vi "SVN_ParseRevisionNumber.vi"(11 "rev str (In)":string) -> (3 "number":i32)   [LabVIEW 2014]
panel:
  out "offset past number":i32
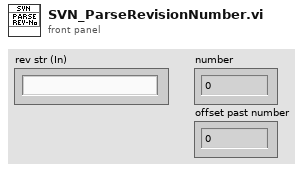
[diagram p1: front panel]
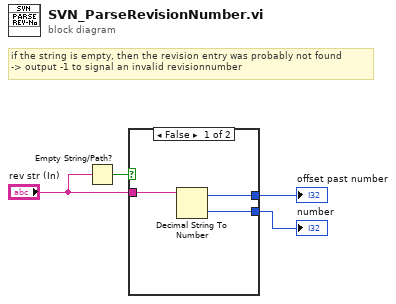
[diagram p0: block diagram]
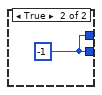
[diagram p2: hidden frame]
diagram:
  # "if the string is empty, then the revision entry was probably not found\n-> output -1 to signal an invalid revisionnumber"
  n1 = Empty String/Path?(string/path="rev str (In)") -> (empty?=w1:bool)
  n2 = case shown="False" w1 {
    tunnel: [w7 w8] -> w4
    tunnel: [w6 w8] -> w3
    tunnel: "rev str (In)" -> [w5 _]
    frame False {
      n3 = Decimal String To Number(string=w5) -> (offset past number=w6:i32, number=w7:i32)  [unwired: 2 in]
    }
    frame True {
      w8 = -1
    }
  }
  "number" <- w4
  "offset past number" <- w3
